vi "Gmail_send.vi"(0 "Attachment - Optional":path, 1 "Body":string, 2 "Subject":string, 3 "CC - Optional":string, 4 "Target address":string, 5 "GMAIL Account Password":string, 6 "GMAIL Account User ID":string) -> ()   [LabVIEW 2016]
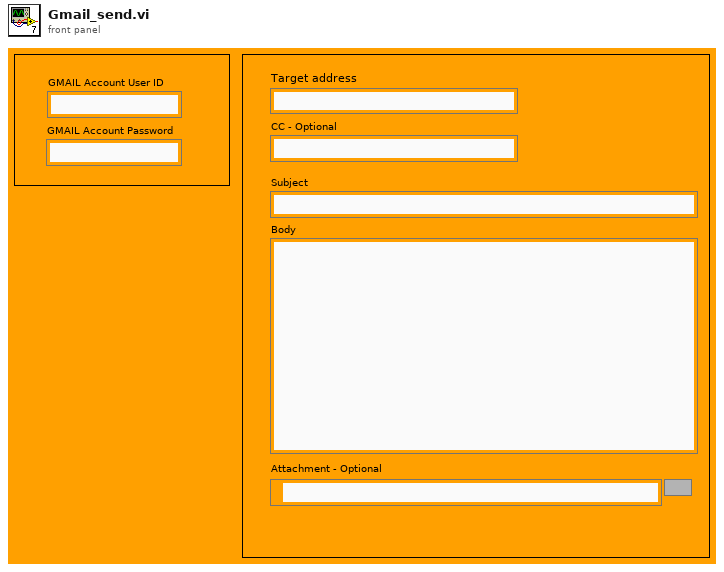
[diagram p1: front panel]
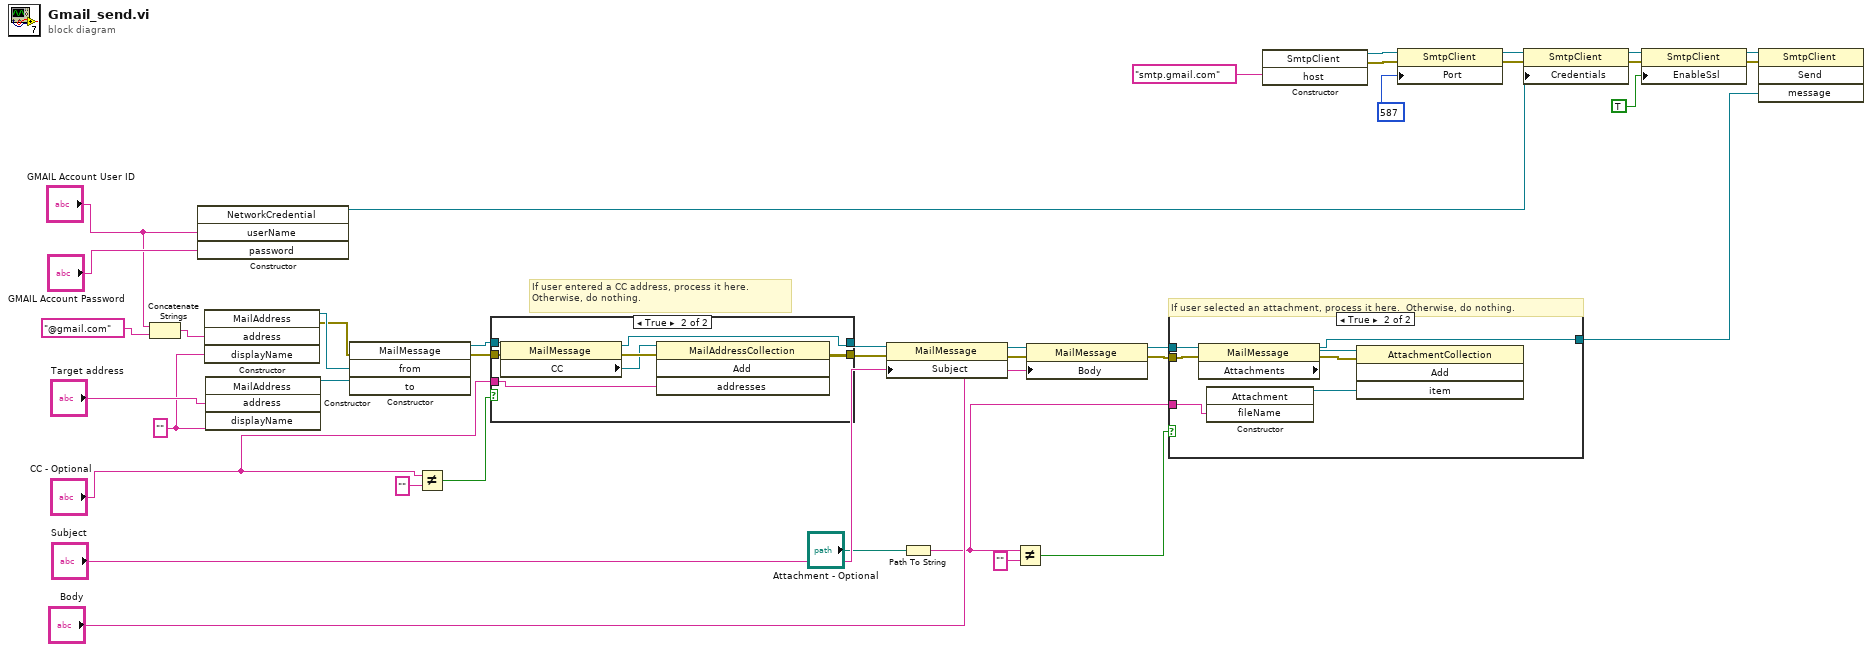
[diagram p0: block diagram]
diagram:
  w1 = "" ("Recipient's Name")
  # "If user selected an attachment, process it here.  Otherwise, do nothing."
  # "If user entered a CC address, process it here.\nOtherwise, do nothing."
  n1 = Concatenate Strings("GMAIL Account User ID", "@gmail.com" ("string")) -> (w3:string)
  n2 = constructor class="NetworkCredential"("userName"="GMAIL Account User ID", "password"="GMAIL Account Password") -> (reference out=w29:refnum<k24>)  [unwired: 3 in, 4 out]
  n3 = constructor class="MailAddress"("address"=w3, "displayName"=w1) -> (reference out=w38:refnum<k24>, error out=w7:errorcluster)  [unwired: 3 in, 3 out]
  n4 = constructor class="MailAddress"("address"="Target address", "displayName"=w1) -> (reference out=w39:refnum<k24>)  [unwired: 3 in, 4 out]
  n5 = constructor class="MailMessage"(error in=w7, "from"=w38, "to"=w39) -> (reference out=w14:refnum<k24>, error out=w13:errorcluster)  [unwired: 2 in, 3 out]
  n6 = Not Equal?(x="CC - Optional", y="") -> (x != y?=w16:bool)
  n7 = case shown="True" w16 {
    tunnel: "CC - Optional" -> [_ w46]
    tunnel: w14 -> [w41 w45]
    tunnel: w13 -> [w40 w44]
    tunnel: [w41 w43] -> w12
    tunnel: [w40 w42] -> w11
    frame False {
    }
    frame True {
      n8 = property class="MailMessage"(reference=w45, error in=w44) -> (reference out=w43:refnum<k24>, error out=w48:errorcluster, "CC"=w47:refnum<k24>)
      n9 = invoke class="MailAddressCollection" method="Add"(reference=w47, error in=w48, "addresses"=w46) -> (error out=w42:errorcluster)  [unwired: 1 in, 3 out]
    }
  }
  n10 = property class="MailMessage"(reference=w12, error in=w11, "Subject"="Subject") -> (reference out=w33:refnum<k24>, error out=w37:errorcluster)
  n11 = Path To String(path="Attachment - Optional") -> (string=w18:string)
  n12 = Not Equal?(x=w18, y="") -> (x != y?=w19:bool)
  n13 = property class="MailMessage"(reference=w33, error in=w37, "Body"="Body") -> (reference out=w22:refnum<k24>, error out=w6:errorcluster)
  n14 = case shown="True" w19 {
    tunnel: w22 -> [w49 w53]
    tunnel: [w49 w52] -> w10
    tunnel: w18 -> [_ w51]
    tunnel: w6 -> [_ w50]
    frame False {
    }
    frame True {
      n15 = property class="MailMessage"(reference=w53, error in=w50) -> (reference out=w52:refnum<k24>, error out=w56:errorcluster, "Attachments"=w54:refnum<k24>)
      n16 = constructor class="Attachment"("fileName"=w51) -> (reference out=w55:refnum<k24>)  [unwired: 3 in, 3 out]
      n17 = invoke class="AttachmentCollection" method="Add"(reference=w54, error in=w56, "item"=w55) -> ()  [unwired: 1 in, 4 out]
    }
  }
  n18 = constructor class="SmtpClient"("host"="smtp.gmail.com" ("Outgoing Mail Server (SMTP)")) -> (reference out=w28:refnum<k24>, error out=w25:errorcluster)  [unwired: 3 in, 2 out]
  n19 = property class="SmtpClient"(reference=w28, error in=w25, "Port"=587) -> (reference out=w27:refnum<k24>, error out=w24:errorcluster)
  n20 = property class="SmtpClient"(reference=w27, error in=w24, "Credentials"=w29) -> (reference out=w26:refnum<k24>, error out=w23:errorcluster)
  n21 = property class="SmtpClient"(reference=w26, error in=w23, "EnableSsl"=TRUE ("Enable SSL")) -> (reference out=w8:refnum<k24>, error out=w9:errorcluster)
  n22 = invoke class="SmtpClient" method="Send"(reference=w8, error in=w9, "message"=w10) -> ()  [unwired: 1 in, 4 out]
